vi "create_systemcheck_devices.vi"(8 "error in (no error)":errorcluster) -> (0 "error out":errorcluster)   [LabVIEW 2017]
doc: "reads settings for each switch in \"SystemDevices.ini\" and creates objects for each of those devices (Pressure Gauges, Temp-Indicators, Temp-Controllers). those objects are stored in a global variable. The global variable stores any object no matter what type"
uses:
  Classes/PrepLineObject/PrepLineObject.lvclass
  global variables.vi
  <vilib>/Utility/config.llb/Read Key (String).vi
  <vilib>/Utility/config.llb/Read Key (I32).vi
  Classes/StatusLog/StatusLog.lvclass
  <vilib>/Utility/config.llb/NI_LVConfig.lvlib
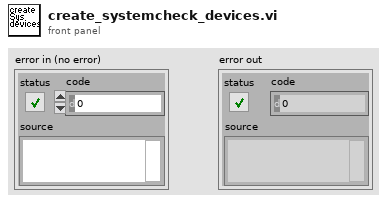
[diagram p1: front panel]
types:
  T1 = typedef "NI_LVConfig.lvlib/Config Data RefNum.ctl" = refnum<k1>
  T2 = typedef "Semaphore RefNum" = refnum<k1>
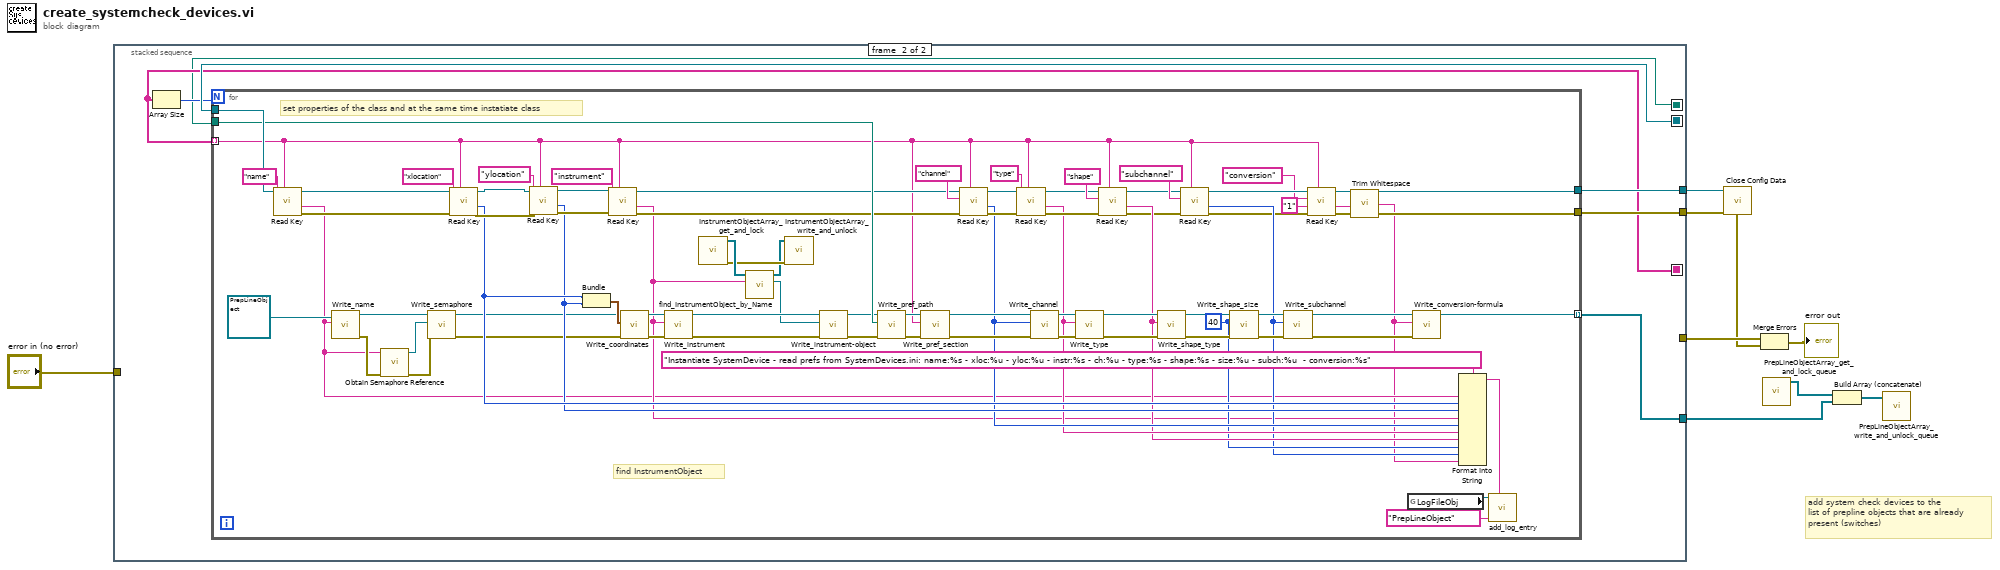
[diagram p0: block diagram]
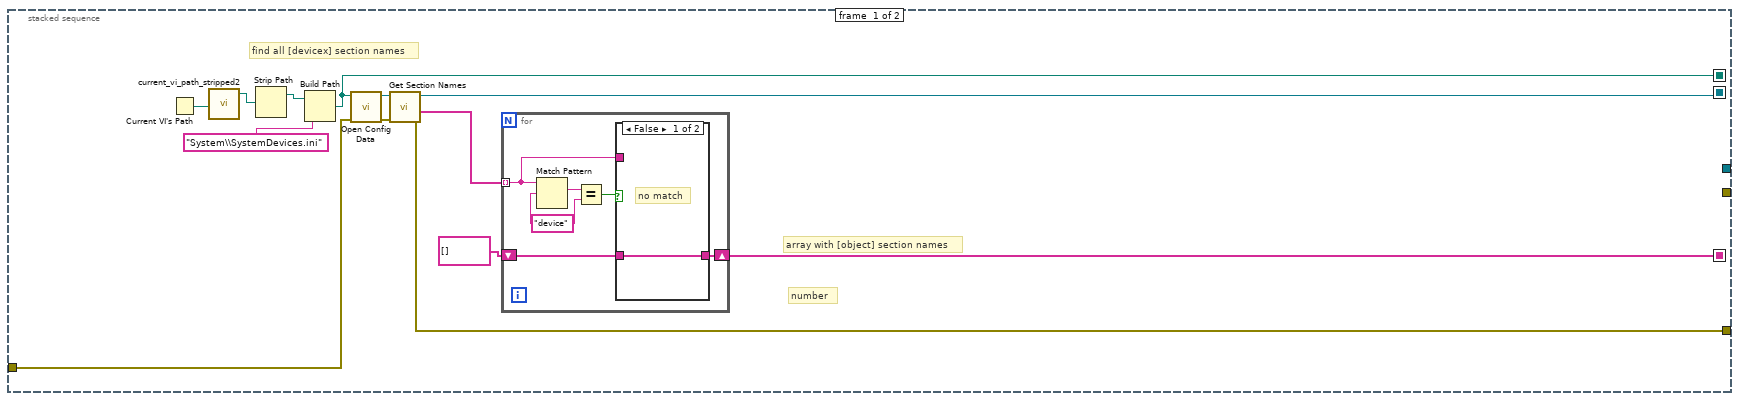
[diagram p2: hidden frame]
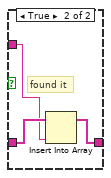
[diagram p3: hidden frame]
diagram:
  # "add system check devices to the\nlist of prepline objects that are already\npresent (switches)"
  n1 = stacked-sequence {
    seq-local: [w18 _] -> [_ w39]
    seq-local: [w14 _] -> [_ w35]
    seq-local: [w13 _] -> [_ w34]
    tunnel: "error in (no error)" -> [w19 _]
    tunnel: [w17 _] -> w8
    tunnel: [_ w38] -> w6
    tunnel: [_ w37] -> w5
    tunnel: [_ w33] -> w3
    frame #0 {
      # "number"
      # "array with [object] section names"
      # "find all [devicex] section names"
      n2 = Current VI's Path() -> (path=w12:path)
      n3 = call "current_vi_path_stripped2.vi"("current VI Path"=w12) -> ("current VI Path stripped out"=w10:path)  [unwired: 3 in, 1 out]
      n4 = Strip Path(path=w10) -> (stripped path=w11:path)  [unwired: 1 out]
      n5 = Build Path(base path=w11, name or relative path="System\\SystemDevices.ini") -> (appended path=w13:path)
      n6 = call <vilib>:"Open Config Data.vi"("error in (no error)"=w19, "configuration file path"=w13) -> ("error out"=w20:errorcluster, "refnum"=w21:T1)  [unwired: 7 in, 1 out]
      n7 = call <vilib>:"Get Section Names.vi"("error in (no error)"=w20, "refnum"=w21) -> ("error out"=w17:errorcluster, "section names"=w16:string[], "refnum out"=w18:T1)  [unwired: 7 in]
      n8 = for {
        tunnel: w16 -> [w25] mode=indexing
        shift-right: [w23] -> w14
        shift-left: string[] [] ("section names") -> [w24]
        w27 = "device" ("regular expression")
        n9 = Match Pattern(string=w25, regular expression=w27) -> (match substring=w28:string)  [unwired: 1 in, 3 out]
        n10 = Equal?(x=w28, y=w27) -> (x = y?=w26:bool)
        n11 = case shown="False" w26 {
          tunnel: w25 -> [_ w31]
          tunnel: [w29 w30] -> w23
          tunnel: w24 -> [w29 w32]
          frame False {
            # "no match"
          }
          frame True {
            # "found it"
            n12 = Insert Into Array(array=w32, new element=w31) -> (w30:string[])  [unwired: 1 in]
          }
        }
      }
    }
    frame #1 {
      n13 = Array Size(array=w35) -> (size(s)=w36:i32)
      n14 = for {
        N: w36 -> [_]
        tunnel: w39 -> [w118]
        tunnel: [w53] -> w38
        tunnel: [w52] -> w37
        tunnel: w35 -> [w51] mode=indexing
        tunnel: w34 -> [w102]
        tunnel: [w47] -> w33 mode=indexing
        w76 = i8 40 ("shape type")
        # "find InstrumentObject"
        # "set properties of the class and at the same time instatiate class"
        n15 = call-poly <vilib>:"Read Key.vi"("section"=w51, "key"="name", "refnum"=w118) -> ("error out"=w110:errorcluster, "value"=w57:string, "refnum out"=w113:T1)  [unwired: 5 in, 1 out]
        n16 = call-dynamic "Write_name.vi"("name"=w57, "PrepLinePictureObjects in"=refnum<class "PrepLineObject.lvclass"> refnum ("PrepLineObject.lvclass")) -> ("error out"=w59:errorcluster, "PrepLinePictureObjects out"=w62:refnum<class "PrepLineObject.lvclass">)  [unwired: 8 in]
        n17 = call <vilib>:"Obtain Semaphore Reference.vi"("error in (no error)"=w59, "name (unnamed)"=w57) -> ("error out"=w58:errorcluster, "semaphore"=w56:T2)  [unwired: 3 in, 1 out]
        n18 = call-dynamic "Write_semaphore.vi"("error in (no error)"=w58, "semaphore"=w56, "PrepLineObject in"=w62) -> ("error out"=w60:errorcluster, "PrepLineObject out"=w61:refnum<class "PrepLineObject.lvclass">)  [unwired: 7 in]
        n19 = call-poly <vilib>:"Read Key.vi"("section"=w51, "error in (no error)"=w110, "key"="xlocation", "refnum"=w113) -> ("error out"=w109:errorcluster, "value"=w81:i32, "refnum out"=w112:T1)  [unwired: 4 in, 1 out]
        n20 = call-poly <vilib>:"Read Key.vi"("section"=w51, "error in (no error)"=w109, "key"="ylocation", "refnum"=w112) -> ("error out"=w108:errorcluster, "value"=w80:i32, "refnum out"=w111:T1)  [unwired: 4 in, 1 out]
        n21 = Bundle("value"=w81, "value"=w80) -> (w107:cluster{"value":i32, "value":i32})  [unwired: 1 in]
        n22 = call-poly <vilib>:"Read Key.vi"("section"=w51, "error in (no error)"=w108, "key"="instrument", "refnum"=w111) -> ("error out"=w94:errorcluster, "value"=w63:string, "refnum out"=w95:T1)  [unwired: 4 in, 1 out]
        n23 = call-dynamic "Write_coordinates.vi"("error in (no error)"=w60, "Coords"=w107, "PrepLinePictureObjects in"=w61) -> ("error out"=w105:errorcluster, "PrepLinePictureObjects out"=w106:refnum<class "PrepLineObject.lvclass">)  [unwired: 7 in]
        n24 = call-dynamic "Write_instrument.vi"("error in (no error)"=w105, "instrument name"=w63, "PrepLinePictureObjects in"=w106) -> ("error out"=w66:errorcluster, "PrepLinePictureObjects out"=w67:refnum<class "PrepLineObject.lvclass">)  [unwired: 7 in]
        n25 = call "InstrumentObjectArray_get_and_lock.vi"() -> ("error out"=w41:errorcluster, "InstrumentsObjects"=w42:refnum<class "instrument.lvclass">[])  [unwired: 10 in]
        n26 = call "find_InstrumentObject_by_Name.vi"("Instrument Name"=w63, "InstrumentObjects"=w42) -> ("found InstrObject out"=w43:refnum<class "instrument.lvclass">, "InstrumentObjects out"=w40:refnum<class "instrument.lvclass">[])  [unwired: 6 in, 2 out]
        n27 = call "InstrumentObjectArray_write_and_unlock.vi"("error in (no error)"=w41, "InstrumentObjects"=w40) -> ()  [unwired: 9 in, 1 out]
        n28 = call-dynamic "Write_instrument-object.vi"("error in (no error)"=w66, "instrument.lvclass"=w43, "PrepLineObject in"=w67) -> ("error out"=w64:errorcluster, "PrepLineObject out"=w65:refnum<class "PrepLineObject.lvclass">)  [unwired: 7 in]
        n29 = call-dynamic "Write_pref_path.vi"("error in (no error)"=w64, "pref path"=w102, "PrepLinePictureObjects in"=w65) -> ("error out"=w103:errorcluster, "PrepLinePictureObjects out"=w104:refnum<class "PrepLineObject.lvclass">)  [unwired: 7 in]
        n30 = call-dynamic "Write_pref_section.vi"("error in (no error)"=w103, "pref section"=w51, "PrepLinePictureObjects in"=w104) -> ("error out"=w91:errorcluster, "PrepLinePictureObjects out"=w92:refnum<class "PrepLineObject.lvclass">)  [unwired: 7 in]
        n31 = call-poly <vilib>:"Read Key.vi"("section"=w51, "error in (no error)"=w94, "key"="channel", "refnum"=w95) -> ("error out"=w101:errorcluster, "value"=w79:i32, "refnum out"=w100:T1)  [unwired: 4 in, 1 out]
        n32 = call-poly <vilib>:"Read Key.vi"("section"=w51, "error in (no error)"=w101, "key"="type", "refnum"=w100) -> ("error out"=w88:errorcluster, "value"=w78:string, "refnum out"=w89:T1)  [unwired: 4 in, 1 out]
        n33 = call-dynamic "Write_channel.vi"("error in (no error)"=w91, "channel"=w79, "PrepLineObject in"=w92) -> ("error out"=w96:errorcluster, "PrepLineObject out"=w97:refnum<class "PrepLineObject.lvclass">)  [unwired: 7 in]
        n34 = call-dynamic "Write_type.vi"("error in (no error)"=w96, "device type"=w78, "PrepLinePictureObjects in"=w97) -> ("error out"=w86:errorcluster, "PrepLinePictureObjects out"=w87:refnum<class "PrepLineObject.lvclass">)  [unwired: 7 in]
        n35 = call-poly <vilib>:"Read Key.vi"("section"=w51, "error in (no error)"=w88, "key"="shape", "refnum"=w89) -> ("error out"=w69:errorcluster, "value"=w77:string, "refnum out"=w70:T1)  [unwired: 4 in, 1 out]
        n36 = call-dynamic "Write_shape_type.vi"("error in (no error)"=w86, "shape type"=w77, "PrepLinePictureObjects in"=w87) -> ("error out"=w84:errorcluster, "PrepLinePictureObjects out"=w85:refnum<class "PrepLineObject.lvclass">)  [unwired: 7 in]
        n37 = call-poly <vilib>:"Read Key.vi"("section"=w51, "error in (no error)"=w69, "key"="subchannel", "refnum"=w70) -> ("error out"=w54:errorcluster, "value"=w68:i32, "refnum out"=w55:T1)  [unwired: 4 in, 1 out]
        n38 = call-dynamic "Write_shape_size.vi"("error in (no error)"=w84, "shape type"=w76, "PrepLinePictureObjects in"=w85) -> ("error out"=w72:errorcluster, "PrepLinePictureObjects out"=w73:refnum<class "PrepLineObject.lvclass">)  [unwired: 7 in]
        n39 = call-dynamic "Write_subchannel.vi"("error in (no error)"=w72, "subchannel"=w68, "PrepLineObject in"=w73) -> ("error out"=w48:errorcluster, "PrepLineObject out"=w49:refnum<class "PrepLineObject.lvclass">)  [unwired: 7 in]
        n40 = call-poly <vilib>:"Read Key.vi"("section"=w51, "error in (no error)"=w54, "default value"="1", "key"="conversion", "refnum"=w55) -> ("error out"=w52:errorcluster, "value"=w46:string, "refnum out"=w53:T1)  [unwired: 3 in, 1 out]
        n41 = call <vilib>:"Trim Whitespace.vi"("string"=w46) -> ("trimmed string"=w45:string)  [unwired: 1 in]
        n42 = global read "global variables.vi" "LogFileObj"() -> (w83:refnum<class "StatusLog.lvclass">)
        n43 = call-dynamic "Write_conversion-formula.vi"("error in (no error)"=w48, "conversion formula"=w45, "PrepLineObject in"=w49) -> ("PrepLineObject out"=w47:refnum<class "PrepLineObject.lvclass">)  [unwired: 7 in, 1 out]
        n44 = Format Into String(format string="Instantiate SystemDevice - read prefs from SystemDevices.ini: name:%s - xloc:%u - yloc:%u - instr:%s - ch:%u - type:%s - shape:%s - size:%u - subch:%u  - conversion:%s", w57, w81, w80, w63, w79, w78, w77, w76, w68, w45) -> (resulting string=w75:string)  [unwired: 2 in, 1 out]
        n45 = call-dynamic "add_log_entry.vi"("new entry"=w75, "log identifiers"="PrepLineObject", "StatusLog in"=w83) -> ()  [unwired: 5 in, 2 out]
      }
    }
  }
  n46 = call <vilib>:"Close Config Data.vi"("error in (no error)"=w5, "refnum"=w6) -> ("error out"=w4:errorcluster)  [unwired: 8 in, 1 out]
  n47 = Merge Errors(w8, w4) -> (→"error out":errorcluster)
  n48 = call "PrepLineObjectArray_get_and_lock_queue.vi"() -> ("PrepLineObjects"=w2:refnum<class "PrepLineObject.lvclass">[])  [unwired: 10 in, 1 out]
  n49 = Build Array (concatenate)(w2, w3) -> (w1:refnum<class "PrepLineObject.lvclass">[])
  n50 = call "PrepLineObjectArray_write_and_unlock_queue.vi"("PrepLineObjArray"=w1) -> ()  [unwired: 10 in, 1 out]
